vi "Value to Range Code.vi"(9 "Manual Range (1.0)":dbl=1.0 min=-999999000000.0 max=999999000000.0 format="%^_7g", 10 "Function (0: DC Volts)":u16(ring) format="%#_2g" items=["DC Volts", "AC Volts", "AC+DC Volts", "2-Wire Resistance", "2-Wire Resistance Low Power", "DC Current", "AC Current", "AC+DC Current", "Diode", "Continuity", "Frequency"]) -> (2 "Range Set Code":string)   [LabVIEW 2020, in "ADCMT7351_ADC.lvlib"]
doc: "This VI convert a value to remote command which set measurement range."
uses:
  ADCMT7351_ADC.lvlib
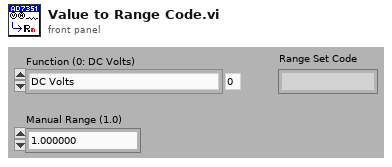
[diagram p1: front panel]
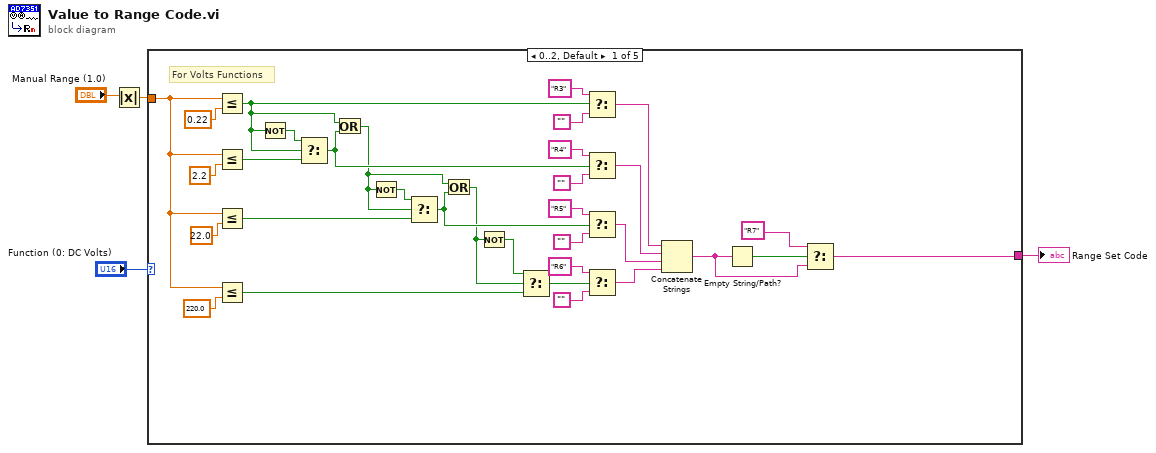
[diagram p0: block diagram]
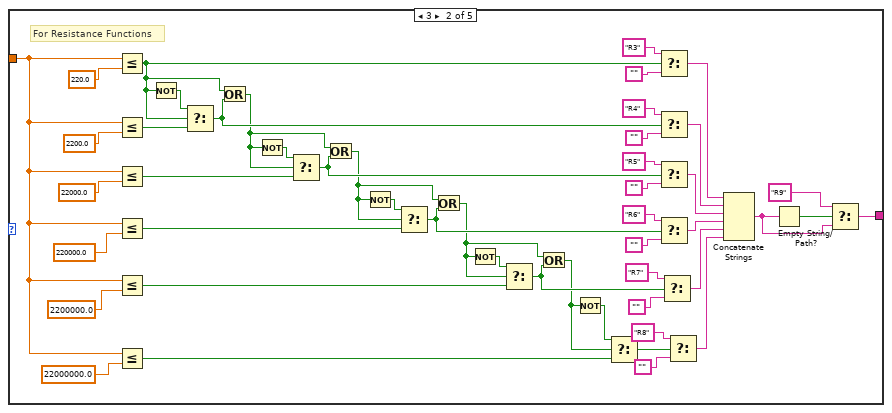
[diagram p2: hidden frame]
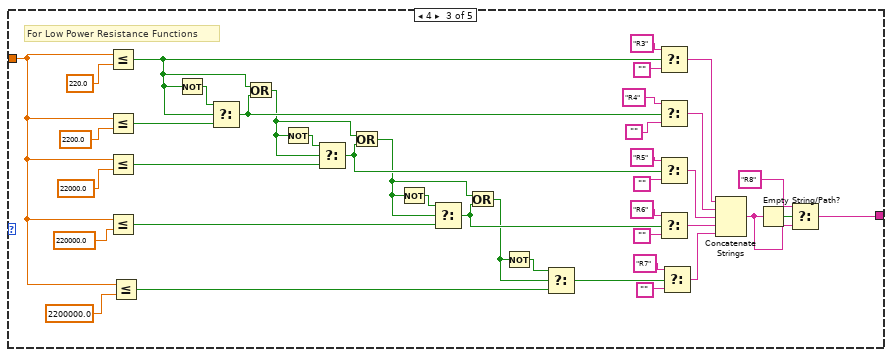
[diagram p3: hidden frame]
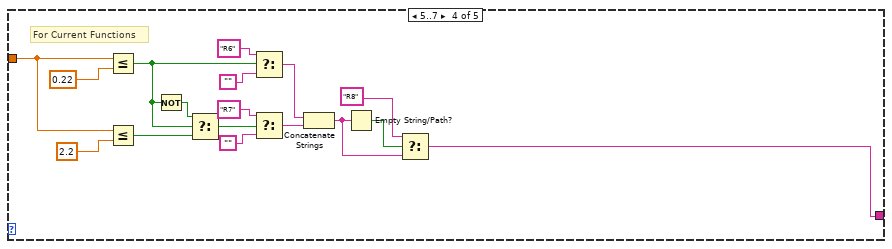
[diagram p4: hidden frame]
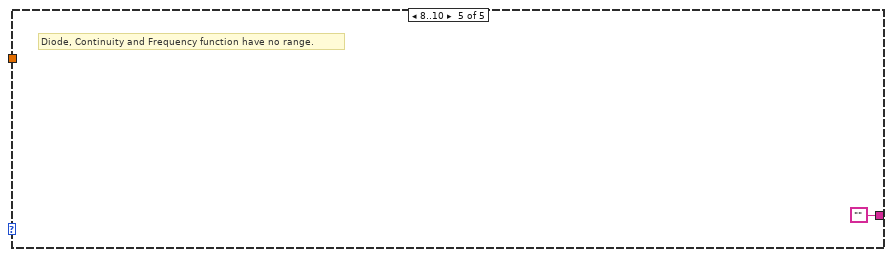
[diagram p5: hidden frame]
diagram:
  n1 = Absolute Value(x="Manual Range (1.0)") -> (abs(x)=w3:dbl)
  n2 = case shown="0..2, Default" "Function (0: DC Volts)" {
    tunnel: w3 -> [w26 w40 w89 w130 _]
    tunnel: [w18 w69 w87 w128 ""] -> w4
    frame 0..2, Default {
      # "For Volts Functions"
      n3 = Less Or Equal?(x=w26, y=0.22) -> (x <= y?=w6:bool)
      n4 = Less Or Equal?(x=w26, y=2.2) -> (x <= y?=w17:bool)
      n5 = Less Or Equal?(x=w26, y=22.0) -> (x <= y?=w14:bool)
      n6 = Less Or Equal?(x=w26, y=220.0) -> (x <= y?=w12:bool)
      n7 = Not(x=w6) -> (.not. x?=w16:bool)
      n8 = Select(t=w16, s=w6, f=w17) -> (s? t:f=w10:bool)
      n9 = Or(x=w6, y=w10) -> (x .or. y?=w7:bool)
      n10 = Not(x=w7) -> (.not. x?=w15:bool)
      n11 = Select(t=w15, s=w7, f=w14) -> (s? t:f=w9:bool)
      n12 = Or(x=w7, y=w9) -> (x .or. y?=w8:bool)
      n13 = Not(x=w8) -> (.not. x?=w13:bool)
      n14 = Select(t=w13, s=w8, f=w12) -> (s? t:f=w11:bool)
      n15 = Select(t="R3", s=w6, f="") -> (s? t:f=w25:string)
      n16 = Select(t="R4", s=w10, f="") -> (s? t:f=w24:string)
      n17 = Select(t="R5", s=w9, f="") -> (s? t:f=w23:string)
      n18 = Select(t="R6", s=w11, f="") -> (s? t:f=w22:string)
      n19 = Concatenate Strings(w25, w24, w23, w22) -> (w19:string)
      n20 = Empty String/Path?(string/path=w19) -> (empty?=w21:bool)
      n21 = Select(t="R7", s=w21, f=w19) -> (s? t:f=w18:string)
    }
    frame 3 {
      # "For Resistance Functions"
      n22 = Less Or Equal?(x=w40, y=220.0) -> (x <= y?=w38:bool)
      n23 = Less Or Equal?(x=w40, y=2200.0) -> (x <= y?=w58:bool)
      n24 = Less Or Equal?(x=w40, y=22000.0) -> (x <= y?=w56:bool)
      n25 = Less Or Equal?(x=w40, y=220000.0) -> (x <= y?=w54:bool)
      n26 = Less Or Equal?(x=w40, y=2200000.0) -> (x <= y?=w50:bool)
      n27 = Less Or Equal?(x=w40, y=22000000.0) -> (x <= y?=w47:bool)
      n28 = Not(x=w38) -> (.not. x?=w59:bool)
      n29 = Select(t=w59, s=w38, f=w58) -> (s? t:f=w53:bool)
      n30 = Or(x=w38, y=w53) -> (x .or. y?=w43:bool)
      n31 = Not(x=w43) -> (.not. x?=w57:bool)
      n32 = Select(t=w57, s=w43, f=w56) -> (s? t:f=w52:bool)
      n33 = Or(x=w43, y=w52) -> (x .or. y?=w42:bool)
      n34 = Not(x=w42) -> (.not. x?=w55:bool)
      n35 = Select(t=w55, s=w42, f=w54) -> (s? t:f=w44:bool)
      n36 = Or(x=w42, y=w44) -> (x .or. y?=w41:bool)
      n37 = Not(x=w41) -> (.not. x?=w51:bool)
      n38 = Select(t=w51, s=w41, f=w50) -> (s? t:f=w49:bool)
      n39 = Or(x=w41, y=w49) -> (x .or. y?=w45:bool)
      n40 = Not(x=w45) -> (.not. x?=w48:bool)
      n41 = Select(t=w48, s=w45, f=w47) -> (s? t:f=w46:bool)
      n42 = Select(t="R3", s=w38, f="") -> (s? t:f=w39:string)
      n43 = Select(t="R4", s=w53, f="") -> (s? t:f=w74:string)
      n44 = Select(t="R5", s=w52, f="") -> (s? t:f=w73:string)
      n45 = Select(t="R6", s=w44, f="") -> (s? t:f=w62:string)
      n46 = Select(t="R7", s=w49, f="") -> (s? t:f=w60:string)
      n47 = Select(t="R8", s=w46, f="") -> (s? t:f=w61:string)
      n48 = Concatenate Strings(w39, w74, w73, w62, w60, w61) -> (w70:string)
      n49 = Empty String/Path?(string/path=w70) -> (empty?=w72:bool)
      n50 = Select(t="R9", s=w72, f=w70) -> (s? t:f=w69:string)
    }
    frame 4 {
      # "For Low Power Resistance Functions"
      n51 = Less Or Equal?(x=w89, y=220.0) -> (x <= y?=w88:bool)
      n52 = Less Or Equal?(x=w89, y=2200.0) -> (x <= y?=w103:bool)
      n53 = Less Or Equal?(x=w89, y=22000.0) -> (x <= y?=w101:bool)
      n54 = Less Or Equal?(x=w89, y=220000.0) -> (x <= y?=w99:bool)
      n55 = Less Or Equal?(x=w89, y=2200000.0) -> (x <= y?=w95:bool)
      n56 = Not(x=w88) -> (.not. x?=w104:bool)
      n57 = Select(t=w104, s=w88, f=w103) -> (s? t:f=w98:bool)
      n58 = Or(x=w88, y=w98) -> (x .or. y?=w92:bool)
      n59 = Not(x=w92) -> (.not. x?=w102:bool)
      n60 = Select(t=w102, s=w92, f=w101) -> (s? t:f=w97:bool)
      n61 = Or(x=w92, y=w97) -> (x .or. y?=w91:bool)
      n62 = Not(x=w91) -> (.not. x?=w100:bool)
      n63 = Select(t=w100, s=w91, f=w99) -> (s? t:f=w93:bool)
      n64 = Or(x=w91, y=w93) -> (x .or. y?=w90:bool)
      n65 = Not(x=w90) -> (.not. x?=w96:bool)
      n66 = Select(t=w96, s=w90, f=w95) -> (s? t:f=w94:bool)
      n67 = Select(t="R3", s=w88, f="") -> (s? t:f=w115:string)
      n68 = Select(t="R4", s=w98, f="") -> (s? t:f=w114:string)
      n69 = Select(t="R5", s=w97, f="") -> (s? t:f=w113:string)
      n70 = Select(t="R6", s=w93, f="") -> (s? t:f=w106:string)
      n71 = Select(t="R7", s=w94, f="") -> (s? t:f=w105:string)
      n72 = Concatenate Strings(w115, w114, w113, w106, w105) -> (w110:string)
      n73 = Empty String/Path?(string/path=w110) -> (empty?=w112:bool)
      n74 = Select(t="R8", s=w112, f=w110) -> (s? t:f=w87:string)
    }
    frame 5..7 {
      # "For Current Functions"
      n75 = Less Or Equal?(x=w130, y=0.22) -> (x <= y?=w129:bool)
      n76 = Less Or Equal?(x=w130, y=2.2) -> (x <= y?=w132:bool)
      n77 = Not(x=w129) -> (.not. x?=w133:bool)
      n78 = Select(t=w133, s=w129, f=w132) -> (s? t:f=w131:bool)
      n79 = Select(t="R6", s=w129, f="") -> (s? t:f=w138:string)
      n80 = Select(t="R7", s=w131, f="") -> (s? t:f=w137:string)
      n81 = Concatenate Strings(w138, w137) -> (w134:string)
      n82 = Empty String/Path?(string/path=w134) -> (empty?=w136:bool)
      n83 = Select(t="R8", s=w136, f=w134) -> (s? t:f=w128:string)
    }
    frame 8..10 {
      # "Diode, Continuity and Frequency function have no range."
    }
  }
  "Range Set Code" <- w4
